vi "Add Tree Nodes.vi"(7 "Root path":string, 8 "Event Types":T1[](array[typedef]), 9 "map ref in":map{string, refnum<vi>}(c390), 10 "DQMH Lib In":refnum<vi>, 11 "Tree Map in":T2) -> (1 "map ref out":map{string, refnum<vi>}(c390), 3 "Tree Map out":T2)   [LabVIEW 2020, in "Panther Dashboard.lvlib"]
uses:
  Panther Dashboard.lvlib
  <vilib>/National Instruments/Tree Map/Tree Map Data.ctl
  Event types--enum.ctl
  <vilib>/National Instruments/Tree Map/Tree Map.lvlib
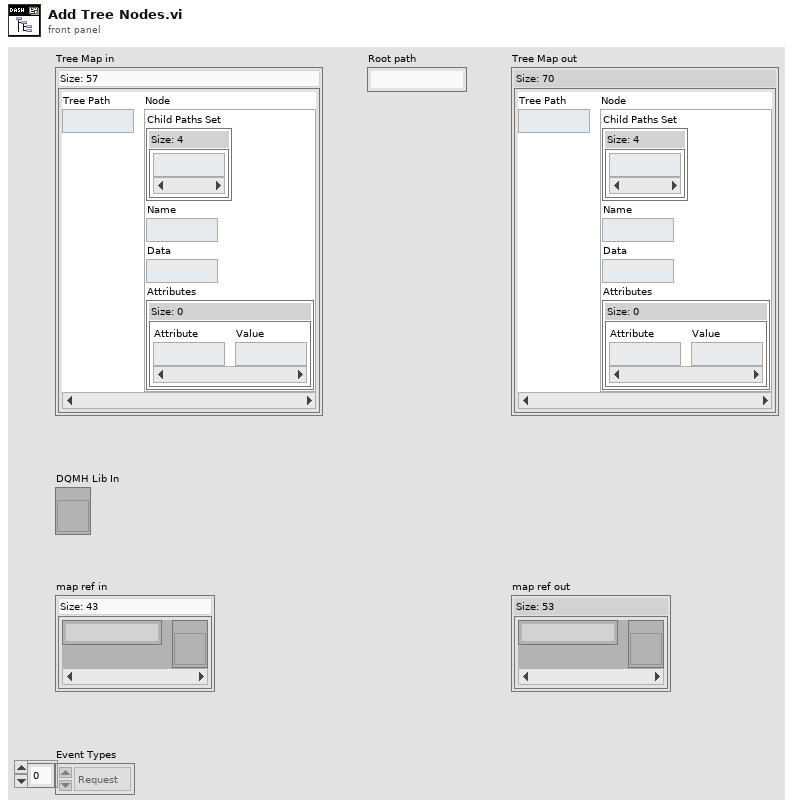
[diagram p1: front panel]
types:
  T1 = typedef "Panther Dashboard.lvlib/Event types--enum.ctl" = enum16{"Request", "Request and Wait for Reply", "Broadcast"}
  T2 = typedef "Tree Map.lvlib/Tree Map Data.ctl" = map{string, cluster{"Child Paths Set":set{string}, "Name":string, "Data":string, "Attributes":map{string, string}}}
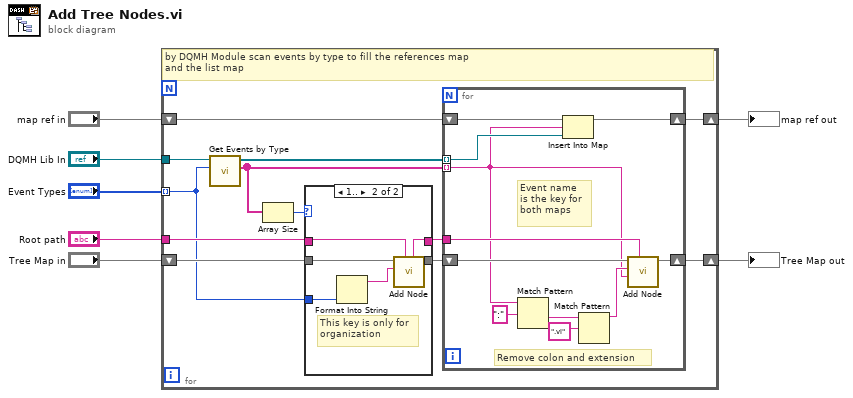
[diagram p0: block diagram]
diagram:
  n1 = for {
    tunnel: "DQMH Lib In" -> [w16]
    tunnel: "Root path" -> [w15]
    tunnel: "Event Types" -> [w10] mode=indexing
    shift-right: [w18] -> w7
    shift-left: "map ref in" -> [w17]
    shift-right: [w14] -> w3
    shift-left: "Tree Map in" -> [w11]
    # "by DQMH Module scan events by type to fill the references map\nand the list map"
    n2 = call "Get Events by Type.vi"("Event type"=w10, "DQMH Module Ref"=w16) -> ("Event Name"=w9:string[], "Event Ref"=w19:refnum<vi>[])  [unwired: 7 in, 1 out]
    n3 = Array Size(array=w9) -> (size(s)=w8:i32)
    n4 = case shown="1.." w8 {
      tunnel: w15 -> [w21 w27]
      tunnel: [w20 w26] -> w13
      tunnel: [w21 w25] -> w12
      tunnel: w11 -> [w20 w24]
      tunnel: w10 -> [_ w22]
      frame 0, Default {
        # "If no Events\nfrom this category \nnot adding\ntag"
      }
      frame 1.. {
        # "This key is only for\norganization"
        n5 = Format Into String(w22) -> (resulting string=w23:string)  [unwired: 3 in, 1 out]
        n6 = call <vilib>:"Add Node.vi"("Parent Path"=w27, "New Node Name"=w23, "Tree Map In"=w24) -> ("Tree Map Out"=w26:T2, "New Node Path"=w25:string)  [unwired: 6 in, 1 out]
      }
    }
    n7 = for {
      tunnel: w12 -> [w38]
      shift-right: [w36] -> w14
      shift-left: w13 -> [w37]
      tunnel: w9 -> [w28] mode=indexing
      shift-right: [w34] -> w18
      shift-left: w17 -> [w35]
      tunnel: w19 -> [w29] mode=indexing
      # "Event name\nis the key for \nboth maps"
      # "Remove colon and extension"
      n8 = Match Pattern(string=w28, regular expression=":") -> (after substring=w31:string)  [unwired: 1 in, 3 out]
      n9 = Insert Into Map(map in=w35, key=w28, value=w29) -> (map out=w34:map{string, refnum<vi>})  [unwired: 2 out]
      n10 = Match Pattern(string=w31, regular expression=".vi") -> (before substring=w30:string)  [unwired: 1 in, 3 out]
      n11 = call <vilib>:"Add Node.vi"("Parent Path"=w38, "Data"=w28, "New Node Name"=w30, "Tree Map In"=w37) -> ("Tree Map Out"=w36:T2)  [unwired: 5 in, 2 out]
    }
  }
  "map ref out" <- w7
  "Tree Map out" <- w3
